vi "Process.CloseAndStop.vi"(8 "error in":errorcluster, 11 "State Variables":T1) -> (0 "error out":errorcluster, 3 "State Variables":T1)   [LabVIEW 2025, in "bus_monitor_server_do.lvlib"]
doc: "Stop all XNET sessions (Incoming and Outgoing).\nStop Async StreamProcess.Main.vi."
uses:
  bus_monitor_server_do.lvlib
  Types/StreamProcess.VIRef.ctl
  Types/StreamProcess.Refs.ctl
  bus_monitor_server/RPC Messages/ni_bus_monitor_api_Session.ctl
  bus_monitor_server/bus_monitor_server.lvlib
  Types/XNET.InitialSettings.ctl
  Types/MainProcess.StateVariables.ctl
  bus_monitor_server/RPC Messages/ni_bus_monitor_api_FrameFilter.ctl
  bus_monitor_server/RPC Messages/ni_bus_monitor_api_DirectionFilter.ctl
  bus_monitor_server/RPC Messages/ni_bus_monitor_api_FilterInfo.ctl
  bus_monitor_server/RPC Messages/ni_bus_monitor_api_FdIsoMode.ctl
  bus_monitor_server/RPC Messages/ni_bus_monitor_api_Termination.ctl
  bus_monitor_server/RPC Messages/ni_bus_monitor_api_CanMode.ctl
  bus_monitor_server/RPC Messages/ni_bus_monitor_api_ConnectSettings.ctl
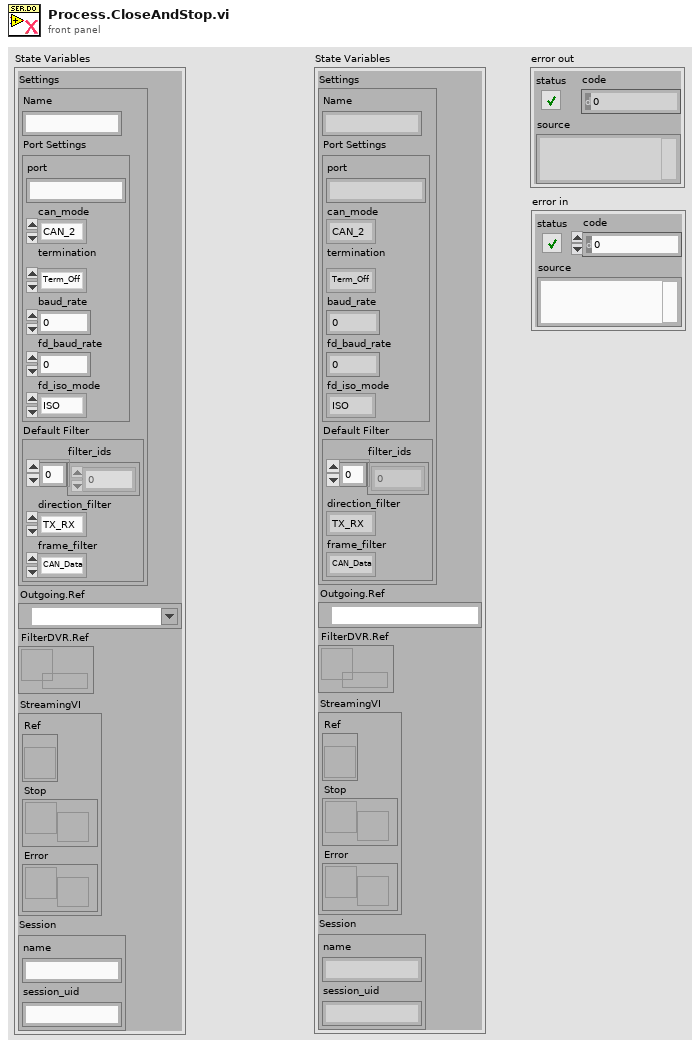
[diagram p1: front panel]
types:
  T1 = typedef "bus_monitor_server_do.lvlib/MainProcess.StateVariables.ctl" = cluster{"Settings":T2, "Outgoing.Ref":refnum<k21>, "FilterDVR.Ref":refnum<data-value>, "StreamingVI":T10, "Session":T12}
  T2 = typedef "bus_monitor_server_do.lvlib/XNET.InitialSettings.ctl" = cluster{"Name":string, "Port Settings":T3, "Default Filter":T7}
  T3 = typedef "bus_monitor_server.lvlib/ni_bus_monitor_api_ConnectSettings.ctl" = cluster{"port":string, "can_mode":T4, "termination":T5, "baud_rate":u64, "fd_baud_rate":u64, "fd_iso_mode":T6}
  T4 = typedef "bus_monitor_server.lvlib/ni_bus_monitor_api_CanMode.ctl" = enum32{"CAN_2", "CAN_FD", "CAN_FD_BRS"}
  T5 = typedef "bus_monitor_server.lvlib/ni_bus_monitor_api_Termination.ctl" = enum32{"Term_Off", "Term_On"}
  T6 = typedef "bus_monitor_server.lvlib/ni_bus_monitor_api_FdIsoMode.ctl" = enum32{"ISO", "Non_ISO", "ISO_Legacy"}
  T7 = typedef "bus_monitor_server.lvlib/ni_bus_monitor_api_FilterInfo.ctl" = cluster{"filter_ids":u32[], "direction_filter":T8, "frame_filter":T9}
  T8 = typedef "bus_monitor_server.lvlib/ni_bus_monitor_api_DirectionFilter.ctl" = enum32{"TX_RX", "RX", "TX"}
  T9 = typedef "bus_monitor_server.lvlib/ni_bus_monitor_api_FrameFilter.ctl" = enum32{"CAN_Data", "CAN_Remote", "CAN_Bus_Error", "CAN_2_Data", "CAN_FD_Data", "CAN_FD_BRS_Data", "J1939_Data", "Delay", "Log_Trigger", "Start_Trigger", "All"}
  T10 = typedef "bus_monitor_server_do.lvlib/StreamProcess.Refs.ctl" = cluster{"Ref":T11, "Stop":refnum<notifier>, "Error":refnum<notifier>}
  T11 = typedef "bus_monitor_server_do.lvlib/StreamProcess.VIRef.ctl" = refnum<vi>
  T12 = typedef "bus_monitor_server.lvlib/ni_bus_monitor_api_Session.ctl" = cluster{"name":string, "session_uid":string}
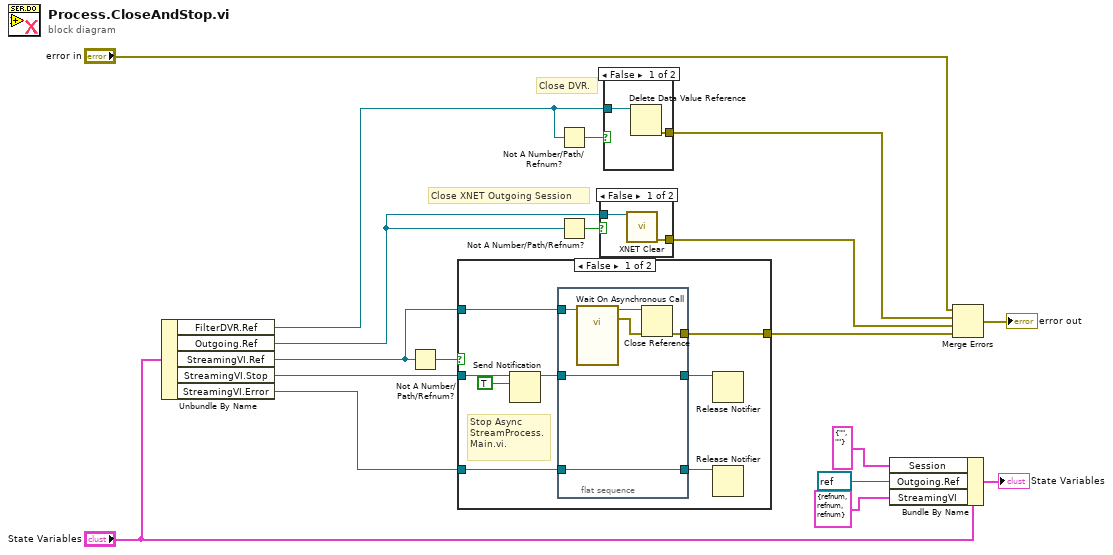
[diagram p0: block diagram]
diagram:
  # "Close XNET Outgoing Session"
  # "Close DVR."
  n1 = Unbundle By Name("State Variables") -> ("FilterDVR.Ref"=w8:refnum<data-value>, "Outgoing.Ref"=w12:refnum<k21>, "StreamingVI.Ref"=w13:T11, "StreamingVI.Stop"=w5:refnum<notifier>, "StreamingVI.Error"=w3:refnum<notifier>)
  n2 = Not A Number/Path/Refnum?(number/path/refnum=w13) -> (NaN/Path/Refnum?=w15:bool)
  n3 = case shown="False" w15 {
    tunnel: w13 -> [w26 _]
    tunnel: [w25 _] -> w17
    tunnel: w5 -> [w23 _]
    tunnel: w3 -> [w19 _]
    frame False {
      # "Stop Async StreamProcess.Main.vi."
      n4 = Send Notification(notification=TRUE, notifier=w23) -> (notifier out=w22:refnum<notifier>)  [unwired: 1 in, 1 out]
      n5 = flat-sequence {
        tunnel: w26 -> [w32]
        tunnel: [w29] -> w25
        tunnel: w22 -> [w28]
        tunnel: [w28] -> w21
        tunnel: [w27] -> w20
        tunnel: w19 -> [w27]
        frame #0 {
          n6 = call-by-ref "Wait On Asynchronous Call"(reference=w32) -> (reference out=w31:T11, error out=w30:errorcluster)  [unwired: 12 in, 1 out]
          n7 = Close Reference(reference=w31, error in (no error)=w30) -> (error out=w29:errorcluster)
        }
      }
      n8 = Release Notifier(notifier=w21) -> ()  [unwired: 2 in, 3 out]
      n9 = Release Notifier(notifier=w20) -> ()  [unwired: 2 in, 3 out]
    }
    frame True {
    }
  }
  n10 = Not A Number/Path/Refnum?(number/path/refnum=w8) -> (NaN/Path/Refnum?=w7:bool)
  n11 = Not A Number/Path/Refnum?(number/path/refnum=w12) -> (NaN/Path/Refnum?=w14:bool)
  n12 = case shown="False" w14 {
    tunnel: w12 -> [w34 _]
    tunnel: [w33 _] -> w16
    frame False {
      n13 = call <vilib>:"XNET Clear.vi"("session in"=w34) -> ("error out"=w33:errorcluster)  [unwired: 14 in]
    }
    frame True {
    }
  }
  n14 = case shown="False" w7 {
    tunnel: w8 -> [w36 _]
    tunnel: [w35 _] -> w6
    frame False {
      n15 = Delete Data Value Reference(data value reference=w36) -> (error out=w35:errorcluster)  [unwired: 1 in, 1 out]
    }
    frame True {
    }
  }
  n16 = Bundle By Name(cluster="State Variables", "Session"=T12 {"name"="", "session_uid"=""}, "Outgoing.Ref"=refnum<k21> refnum, "StreamingVI"=T10 {"Ref"=refnum, "Stop"=refnum, "Error"=refnum}) -> (→"State Variables":T1)
  n17 = Merge Errors("error in", w6, w16, w17) -> (→"error out":errorcluster)
